vi "PWM Data Analysis - CB.vi"(0 "Analysis Leg":i32, 5 "Active Leg":i32, 7 "Duty Cycle":i32=25, 9 "Waveform":waveform(dbl)[](array[waveform])) -> (10 "Result (Boolean)":bool, 15 "Message":string)   [LabVIEW 2022 SP3]
uses:
  <vilib>/measure/mascope.llb/Pulse Measurements 1 chan.vi
  <vilib>/measure/madcrms.llb/Basic Averaged DC-RMS for 1 Chan.vi
  <vilib>/measure/NI_MAPro.lvlib
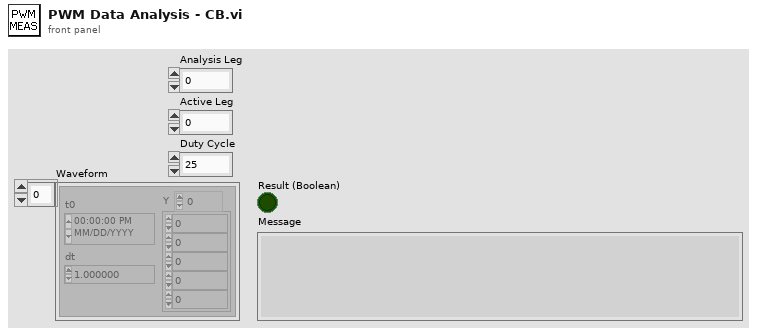
[diagram p1: front panel]
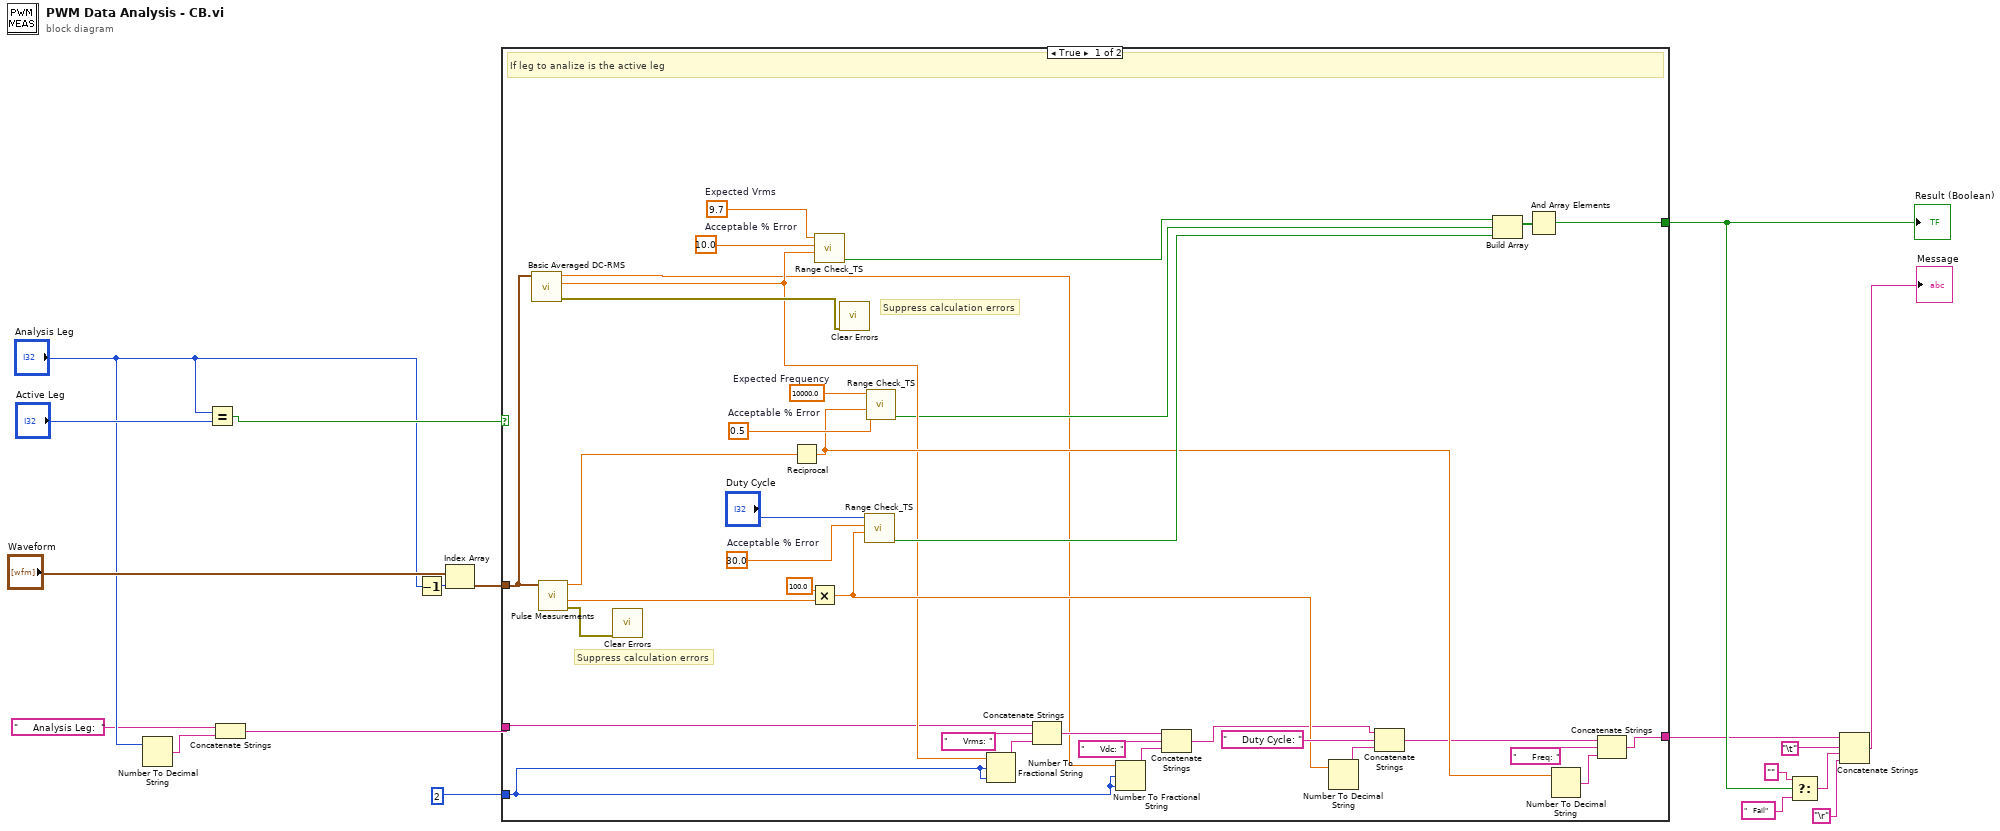
[diagram p0: block diagram]
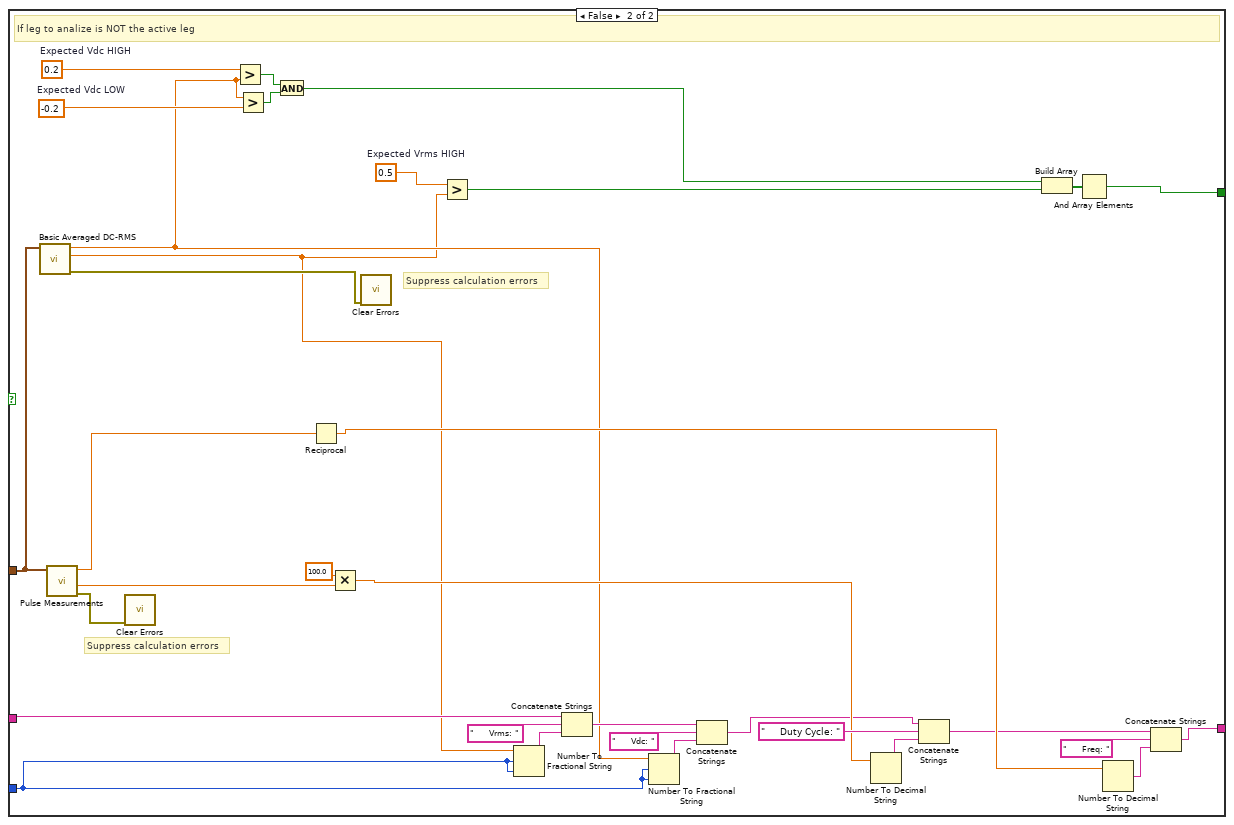
[diagram p2: hidden frame]
diagram:
  n1 = Number To Decimal String(number="Analysis Leg") -> (decimal integer string=w1:string)  [unwired: 1 in]
  n2 = Equal?(x="Analysis Leg", y="Active Leg") -> (x = y?=w5:bool)
  n3 = Concatenate Strings("     Analysis Leg:  ", w1) -> (w2:string)
  n4 = Decrement(x="Analysis Leg") -> (x-1=w18:i32)
  n5 = Index Array(array="Waveform", index=w18) -> (element=w14:waveform(dbl))
  n6 = case shown="True" w5 {
    tunnel: w14 -> [w37 w74]
    tunnel: [w31 w71] -> w10
    tunnel: [w20 w58] -> w9
    tunnel: w2 -> [w22 w60]
    tunnel: 2 -> [w19 w57]
    frame True {
      w25 = 10.0  # Acceptable % Error
      w24 = 9.7  # Expected Vrms
      w46 = 30.0  # Acceptable % Error
      w47 = 0.5  # Acceptable % Error
      w42 = 10000.0  # Expected Frequency
      # "Suppress calculation errors"
      # "Suppress calculation errors"
      # "If leg to analize is the active leg"
      n7 = call-poly <vilib>:"Basic Averaged DC-RMS.vi"("signal in"=w37) -> ("error out"=w38:errorcluster, "RMS value"=w33:dbl, "DC value"=w23:dbl)  [unwired: 7 in, 1 out]
      n8 = call-poly <vilib>:"Pulse Measurements.vi"("signal in"=w37) -> ("error out"=w48:errorcluster, "duty cycle"=w50:dbl, "period"=w49:dbl)  [unwired: 6 in, 2 out]
      n9 = call <vilib>:"Clear Errors.vi"("error in (no error)"=w48) -> ()  [unwired: 5 in, 2 out]
      n10 = Reciprocal(x=w49) -> (1/x=w39:dbl)
      n11 = Multiply(x=100.0, y=w50) -> (x*y=w43:dbl)
      n12 = call "Range Check_TS.vi"("Actual Value"=w33, "Acceptable% Error"=w25, "Expected Value"=w24) -> ("Result (Boolean)"=w36:bool)  [unwired: 6 in, 2 out]
      n13 = call <vilib>:"Clear Errors.vi"("error in (no error)"=w38) -> ()  [unwired: 5 in, 2 out]
      n14 = call "Range Check_TS.vi"("Actual Value"=w43, "Acceptable% Error"=w46, "Expected Value"="Duty Cycle") -> ("Result (Boolean)"=w51:bool)  [unwired: 6 in, 2 out]
      n15 = call "Range Check_TS.vi"("Actual Value"=w39, "Acceptable% Error"=w47, "Expected Value"=w42) -> ("Result (Boolean)"=w32:bool)  [unwired: 6 in, 2 out]
      n16 = Number To Fractional String(number=w33, width (-)=w19, precision (6)=w19) -> (F-format string=w35:string)  [unwired: 1 in]
      n17 = Concatenate Strings(w22, "     Vrms: " ("string"), w35) -> (w27:string)
      n18 = Number To Fractional String(number=w23, width (-)=w19, precision (6)=w19) -> (F-format string=w29:string)  [unwired: 1 in]
      n19 = Concatenate Strings(w27, "     Vdc: " ("string"), w29) -> (w21:string)
      n20 = Number To Decimal String(number=w43) -> (decimal integer string=w44:string)  [unwired: 1 in]
      n21 = Concatenate Strings(w21, "     Duty Cycle: " ("string"), w44) -> (w28:string)
      n22 = Build Array(w36, w32, w51) -> (w52:bool[])
      n23 = And Array Elements(Boolean array=w52) -> (logical AND=w31:bool)
      n24 = Number To Decimal String(number=w39) -> (decimal integer string=w40:string)  [unwired: 1 in]
      n25 = Concatenate Strings(w28, "     Freq: " ("string"), w40) -> (w20:string)
    }
    frame False {
      w56 = 0.5  # Expected Vrms HIGH
      w65 = -0.2  # Expected Vdc LOW
      w66 = 0.2  # Expected Vdc HIGH
      # "Suppress calculation errors"
      # "Suppress calculation errors"
      # "If leg to analize is NOT the active leg"
      n26 = call-poly <vilib>:"Basic Averaged DC-RMS.vi"("signal in"=w74) -> ("error out"=w75:errorcluster, "RMS value"=w55:dbl, "DC value"=w61:dbl)  [unwired: 7 in, 1 out]
      n27 = call-poly <vilib>:"Pulse Measurements.vi"("signal in"=w74) -> ("error out"=w82:errorcluster, "duty cycle"=w84:dbl, "period"=w83:dbl)  [unwired: 6 in, 2 out]
      n28 = call <vilib>:"Clear Errors.vi"("error in (no error)"=w82) -> ()  [unwired: 5 in, 2 out]
      n29 = Greater?(x=w66, y=w61) -> (0:w64:bool)
      n30 = Greater?(x=w61, y=w65) -> (0:w63:bool)
      n31 = And(x=w64, y=w63) -> (x .and. y?=w62:bool)
      n32 = Reciprocal(x=w83) -> (1/x=w76:dbl)
      n33 = Multiply(x=100.0, y=w84) -> (x*y=w79:dbl)
      n34 = call <vilib>:"Clear Errors.vi"("error in (no error)"=w75) -> ()  [unwired: 5 in, 2 out]
      n35 = Greater?(x=w56, y=w55) -> (0:w54:bool)
      n36 = Number To Fractional String(number=w55, width (-)=w57, precision (6)=w57) -> (F-format string=w73:string)  [unwired: 1 in]
      n37 = Concatenate Strings(w60, "     Vrms: " ("string"), w73) -> (w67:string)
      n38 = Number To Fractional String(number=w61, width (-)=w57, precision (6)=w57) -> (F-format string=w69:string)  [unwired: 1 in]
      n39 = Concatenate Strings(w67, "     Vdc: " ("string"), w69) -> (w59:string)
      n40 = Number To Decimal String(number=w79) -> (decimal integer string=w80:string)  [unwired: 1 in]
      n41 = Concatenate Strings(w59, "     Duty Cycle: " ("string"), w80) -> (w68:string)
      n42 = Build Array(w62, w54) -> (w85:bool[])
      n43 = And Array Elements(Boolean array=w85) -> (logical AND=w71:bool)
      n44 = Number To Decimal String(number=w76) -> (decimal integer string=w77:string)  [unwired: 1 in]
      n45 = Concatenate Strings(w68, "     Freq: " ("string"), w77) -> (w58:string)
    }
  }
  "Result (Boolean)" <- w10
  n46 = Select(t="" ("string"), s=w10, f="   Fail" ("string")) -> (s? t:f=w11:string)
  n47 = Concatenate Strings(w9, "\t", w11, "\r") -> (→"Message":string)
